vi "CANOpen Duplicate Device Node.vi"(8 "error in (no error)":errorcluster, 11 "Node Ptr":u64 format="%.0x") -> (0 "error out":errorcluster)   [LabVIEW 2013, in "CANOpen Addon Custom Device.lvlib"]
uses:
  CANOpen Addon Custom Device.lvlib
  <vilib>/NI Veristand/Custom Device API/Custom Device API.lvlib
panel:
  in  "Tag":string
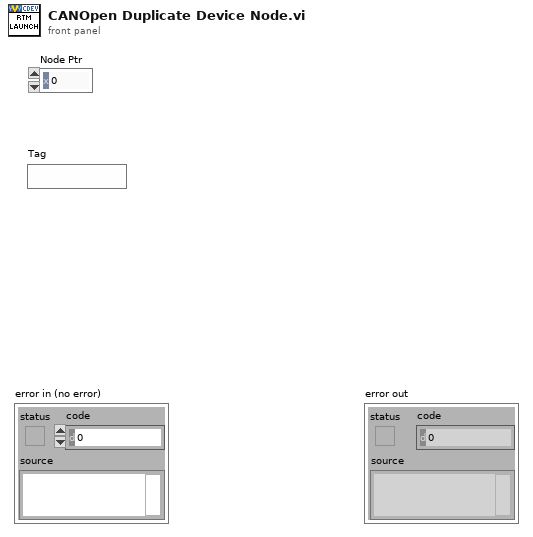
[diagram p1: front panel]
types:
  T1 = typedef "Custom Device API.lvlib/Custom Device Item Ref.ctl" = u64
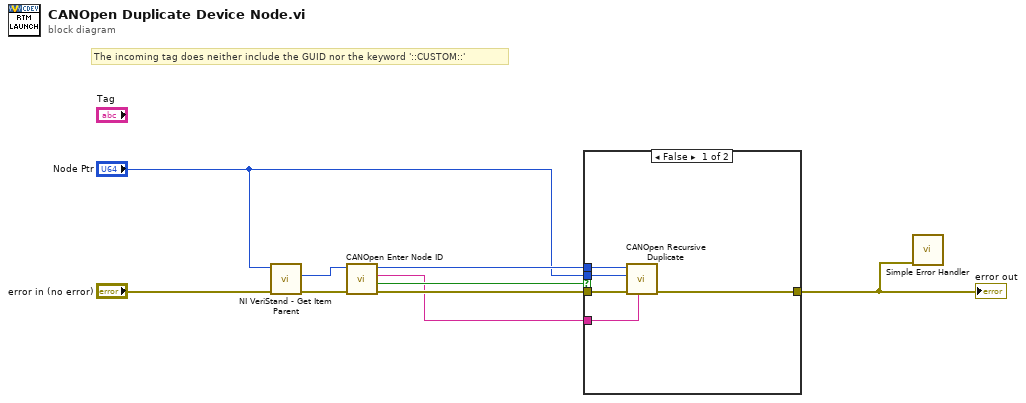
[diagram p0: block diagram]
diagram:
  # "The incoming tag does neither include the GUID nor the keyword '::CUSTOM::'"
  n1 = call <vilib>:"NI VeriStand - Get Item Parent.vi"("error in (no error)"="error in (no error)", "Item Ref in"="Node Ptr") -> ("error out"=w8:errorcluster, "Parent Ref"=w7:T1)  [unwired: 6 in, 2 out]
  n2 = call "CANOpen Enter Node ID.vi"("error in (no error)"=w8, "Node Ptr"=w7) -> ("error out"=w6:errorcluster, "Cancelled?"=w5:bool, "Node ID Out"=w2:string, "Item Ref out"=w4:T1)  [unwired: 5 in, 1 out]
  n3 = case shown="False" w5 {
    tunnel: w6 -> [w14 w15]
    tunnel: [w13 w15] -> w1
    tunnel: w4 -> [w12 _]
    tunnel: "Node Ptr" -> [w11 _]
    tunnel: w2 -> [w10 _]
    frame False {
      n4 = call "CANOpen Recursive Duplicate.vi"("Node ID Name"=w10, "error in (no error)"=w14, "Node Ptr"=w11, "New Node Ptr"=w12) -> ("error out"=w13:errorcluster)  [unwired: 7 in]
    }
    frame True {
    }
  }
  "error out" <- w1
  n5 = call <vilib>:"Simple Error Handler.vi"("error in (no error)"=w1) -> ()  [unwired: 4 in, 5 out]
